vi "DN4_BfdCntr_PwMeterRead.vi"(8 "error in (no error)":errorcluster, 10 "stop?":bool, 11 "Task ID":u32) -> (0 "error out":errorcluster, 1 "stopped":bool, 2 "data":cluster{"high period":dbl, "low period":dbl}[][](array[cluster]), 3 "Task Out ID":u32)   [LabVIEW 2009]
uses:
  Windows/System32/AdvLvDaq.dll
panel:
  out "status":bool
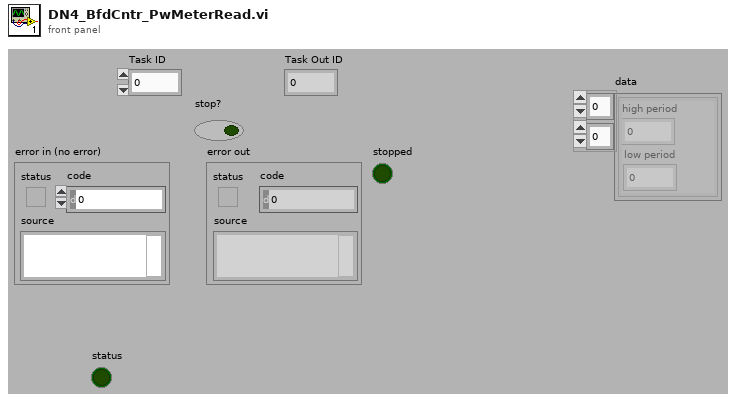
[diagram p1: front panel]
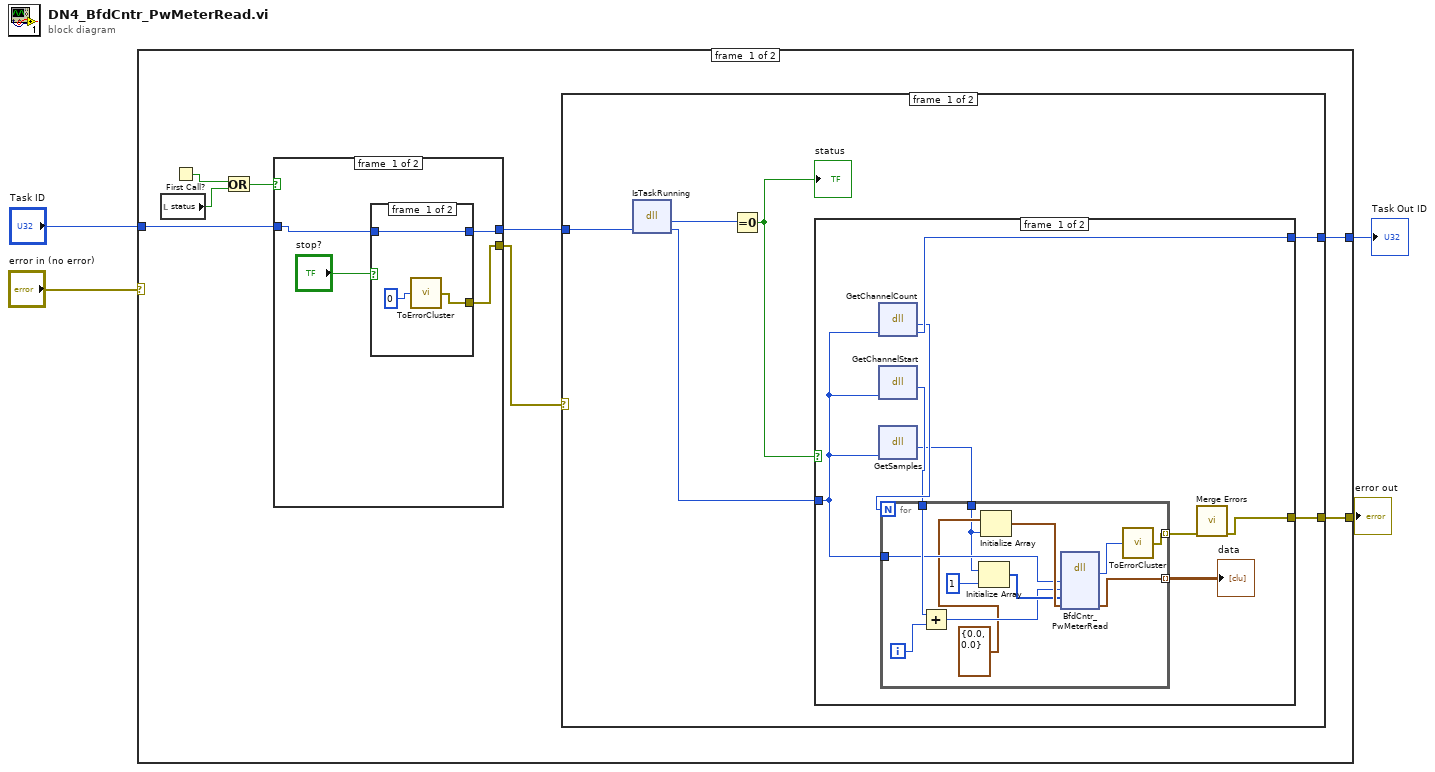
[diagram p0: block diagram]
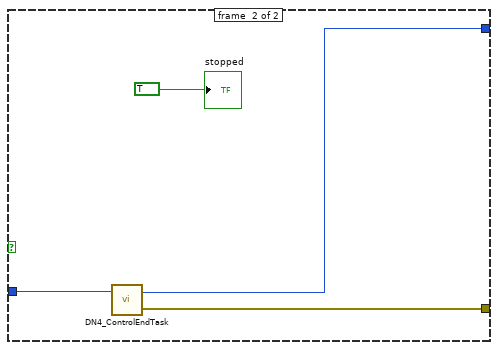
[diagram p2: hidden frame]
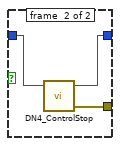
[diagram p4: hidden frame]
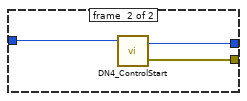
[diagram p5: hidden frame]
diagram:
  n1 = case shown="No Error" "error in (no error)" {
    selector: "error in (no error)" -> [_ w58]
    tunnel: "Task ID" -> [w9 w59]
    tunnel: [w6 w58] -> w2
    tunnel: [w5 w59] -> w1
    frame #0 {
      n2 = local read "status"() -> (w12:bool)
      n3 = First Call?() -> (First Call?: T/F=w11:bool)
      n4 = Or(x=w11, y=w12) -> (x .or. y?=w10:bool)
      n5 = case shown="True" w10 {
        tunnel: w9 -> [w47 w57]
        tunnel: [w46 w56] -> w8
        tunnel: [w45 w55] -> w7
        frame #0 {
          n6 = case shown="True" "stop?" {
            tunnel: w47 -> [w50 w54]
            tunnel: [w49 w53] -> w45
            tunnel: [w50 w52] -> w46
            frame #0 {
              n7 = call <userlib>:"ToErrorCluster.vi"("error code"=0) -> ("error out"=w49:errorcluster)
            }
            frame #1 {
              n8 = call <userlib>:"DN4_ControlStop.vi"("Task ID"=w54) -> ("error out"=w53:errorcluster, "Task ID"=w52:u32)  [unwired: 1 in, 2 out]
            }
          }
        }
        frame #1 {
          n9 = call <userlib>:"DN4_ControlStart.vi"("Task ID"=w57) -> ("error out"=w55:errorcluster, "Task ID"=w56:u32)  [unwired: 1 in, 1 out]
        }
      }
      n10 = case shown="No Error" w7 {
        selector: w7 -> [_ w43]
        tunnel: w8 -> [w18 w44]
        tunnel: [w14 w43] -> w6
        tunnel: [w13 w44] -> w5
        frame #0 {
          n11 = dll-call lib="C:/Windows/System32/AdvLvDaq.dll" fn="IsTaskRunning"("taskId"=w18) -> ("return type"=w17:i8, "taskId"=w15:u32)  [unwired: 3 in, 2 out]
          n12 = Equal To 0?(x=w17) -> (x = 0?=w16:bool)
          "status" <- w16
          n13 = case shown="False" w16 {
            tunnel: w15 -> [w22 w41]
            tunnel: [w20 w40] -> w14
            tunnel: [w26 w39] -> w13
            frame #0 {
              n14 = dll-call lib="C:/Windows/System32/AdvLvDaq.dll" fn="GetChannelCount"("taskId"=w22) -> ("return type"=w25:i32, "taskId"=w26:u32)  [unwired: 3 in, 2 out]
              n15 = dll-call lib="C:/Windows/System32/AdvLvDaq.dll" fn="GetChannelStart"("taskId"=w22) -> ("return type"=w24:i32)  [unwired: 4 in, 2 out]
              n16 = dll-call lib="C:/Windows/System32/AdvLvDaq.dll" fn="GetSamples"("taskId"=w22) -> ("return type"=w23:i32)  [unwired: 4 in, 2 out]
              n17 = for {
                N: w25 -> [_]
                tunnel: w24 -> [w37]
                tunnel: w23 -> [w27]
                tunnel: w22 -> [w32]
                tunnel: [w30] -> w21 mode=indexing
                tunnel: [w28] -> w19 mode=indexing
                i -> [w38]
                n18 = Add(x=w37, y=w38) -> (x+y=w33:i32)
                n19 = Initialize Array(w27, 1) -> (w34:i32[])
                n20 = Initialize Array(cluster{dbl, dbl} {0.0, 0.0}, w27) -> (w35:cluster{dbl, dbl}[])
                n21 = dll-call lib="C:/Windows/System32/AdvLvDaq.dll" fn="BfdCntr_PwMeterRead"("taskId"=w32, "cntr"=w33, "count"=w34, "data"=w35) -> ("return type"=w31:i32, "data"=w28:cluster{dbl, dbl}[])  [unwired: 5 in, 3 out]
                n22 = call <userlib>:"ToErrorCluster.vi"("error code"=w31) -> ("error out"=w30:errorcluster)
              }
              "data" <- w19
              n23 = call <vilib>:"Merge Errors.vi"("error array in"=w21) -> ("error out"=w20:errorcluster)  [unwired: 3 in, 3 out]
            }
            frame #1 {
              n24 = call <userlib>:"DN4_ControlEndTask.vi"("Task ID"=w41) -> ("error out"=w40:errorcluster, "Task ID"=w39:u32)  [unwired: 1 in]
              "stopped" <- TRUE
            }
          }
        }
        frame #1 {
        }
      }
    }
    frame #1 {
    }
  }
  "Task Out ID" <- w1
  "error out" <- w2
